vi "Magazine_Teleop.vi"(11 "Joystick_Out":T1) -> ()   [LabVIEW 2020]
uses:
  Utility VIs/Joystick_Controls.ctl
  Subsystems/Magazine/Magazine_Cluster.ctl
  Subsystems/Magazine/Magazine_Control_States.ctl
  Globals/Magazine_Globals.vi
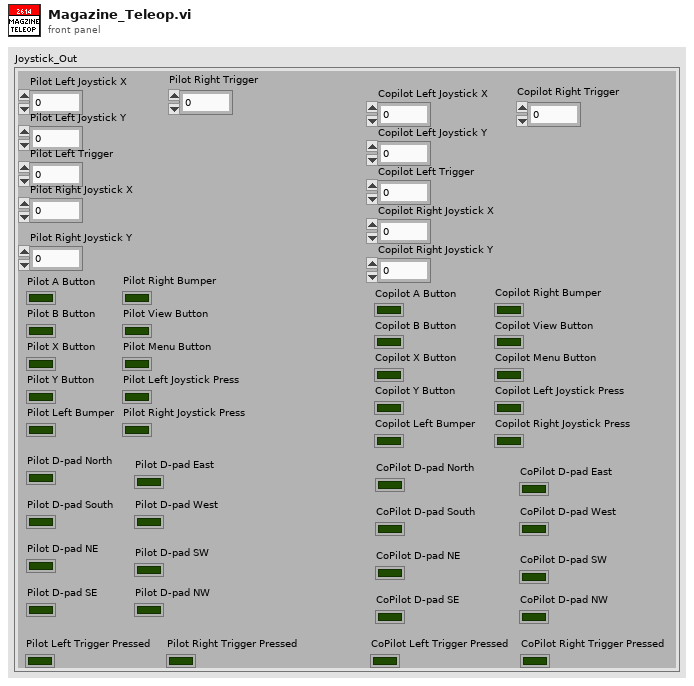
[diagram p1: front panel]
types:
  T1 = typedef "Joystick_Controls.ctl" = cluster{"Pilot Left Joystick X":dbl, "Pilot Left Joystick Y":dbl, "Pilot A Button":bool, "Pilot B Button":bool, "Pilot X Button":bool, "Pilot Y Button":bool, "Pilot Left Bumper":bool, "Pilot Right Bumper":bool, "Pilot View Button":bool, "Pilot Menu Button":bool, "Pilot Left Joystick Press":bool, "Pilot Right Joystick Press":bool, "Pilot Left Trigger":dbl, "Pilot Right Joystick X":dbl, "Pilot Right Joystick Y":dbl, "Pilot Right Trigger":dbl, "Copilot Left Joystick X":dbl, "Copilot Left Joystick Y":dbl, "Copilot A Button":bool, "Copilot B Button":bool, "Copilot X Button":bool, "Copilot Y Button":bool, "Copilot Left Bumper":bool, "Copilot Right Bumper":bool, "Copilot View Button":bool, "Copilot Menu Button":bool, "Copilot Left Joystick Press":bool, "Copilot Right Joystick Press":bool, "Copilot Left Trigger":dbl, "Copilot Right Joystick X":dbl, "Copilot Right Joystick Y":dbl, "Copilot Right Trigger":dbl, "Pilot D-pad North":bool, "Pilot D-pad South":bool, "Pilot D-pad East":bool, "Pilot D-pad West":bool, "Pilot D-pad NE ":bool, "Pilot D-pad SE":bool, "Pilot D-pad SW":bool, "Pilot D-pad NW":bool, "CoPilot D-pad North":bool, "CoPilot D-pad South":bool, "CoPilot D-pad East":bool, "CoPilot D-pad West":bool, "CoPilot D-pad NE":bool, "CoPilot D-pad SE":bool, "CoPilot D-pad SW":bool, "CoPilot D-pad NW":bool, "Pilot Left Trigger Pressed":bool, "Pilot Right Trigger Pressed":bool, "CoPilot Left Trigger Pressed":bool, "CoPilot Right Trigger Pressed":bool}
  T2 = typedef "Magazine_Cluster.ctl" = cluster{"Control_States":T3, "Manual_Magazine":dbl, "Load_Magazine":bool, "Firing_Magazine":bool}
  T3 = typedef "Magazine_Control_States.ctl" = enum16{"No-Op", "Manual_Control", "Load", "Firing"}
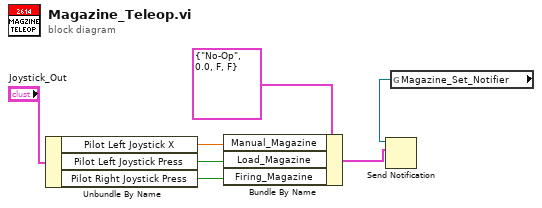
[diagram p0: block diagram]
diagram:
  n1 = Unbundle By Name("Joystick_Out") -> ("Pilot Left Joystick X"=w6:dbl, "Pilot Left Joystick Press"=w2:bool, "Pilot Right Joystick Press"=w1:bool)
  n2 = Bundle By Name(cluster=T2 {"Control_States"=enum."No-Op", "Manual_Magazine"=0.0, "Load_Magazine"=FALSE, "Firing_Magazine"=FALSE}, "Manual_Magazine"=w6, "Load_Magazine"=w2, "Firing_Magazine"=w1) -> (w3:T2)
  n3 = global read "Magazine_Globals.vi" "Magazine_Set_Notifier"() -> (w7:refnum<notifier>)
  n4 = Send Notification(notification=w3, notifier=w7) -> ()  [unwired: 1 in, 2 out]
